vi "CANOpen_Get Section References by GUID for NMT.vi"(7 "Nodes":T2[](array[typedef]) {"NMT"."Node init static SDO state" items=["start remote node"=1, "enter pre-operational"=128]; "NMT"."Node run state" items=["start remote node"=1, "stop remote node"=2, "enter pre-operational"=128, "reset node"=129, "reset communication"=130]; "Dynamic SDOs"."Block Data" format="%.0x"; "RPDOs"."PDO Channel" items=["PDO 1", "PDO 2", "PDO 3", "PDO 4"]; "RPDOs"."Parameters"."Bit Offset" max=8 step=1; "RPDOs"."Parameters"."Byte Offset" max=8 step=1; "TPDOs"."PDO Channel" items=["PDO 1", "PDO 2", "PDO 3", "PDO 4"]; "TPDOs"."Parameters"."Bit Offset" max=8 step=1; "TPDOs"."Parameters"."Byte Offset" max=8 step=1; "SDOs"."Block Data" format="%.0x"}, 8 "error in (no error)":errorcluster, 10 "Node Refs":T1[](array[typedef]) format="%.0x", 11 "Device Ref":T1 format="%.0x") -> (0 "error out":errorcluster, 2 "Data References":T11 {"Hardware Output"."Channel Pairs"."Chan Refs"."Data Reference" format="%.0x"; "Hardware Input"."Channel Pairs"."Chan Refs" format="%.0x"}, 3 "Device Ref out":T1=18446744073709551615 format="%.0x")   [LabVIEW 2013, in "CANOpen Addon Custom Device.lvlib"]
uses:
  CANOpen Addon Custom Device.lvlib
  <vilib>/NI Veristand/Custom Device API/Custom Device Item Ref.ctl
  CANOpen_VS Status Management Data Refs.ctl
  Async VIs/CANOpen_Main/SubVIs/CanOpen_NMT_HWOut_ChannelPairs.ctl
  <vilib>/NI Veristand/Custom Device API/Block Data Reference.ctl
  <vilib>/NI Veristand/Custom Device API/Data Reference.ctl
  Async VIs/CANOpen_Main/SubVIs/CanOpen_NMT_HWIn_ChannelPairs.ctl
  CANOpen_Node Message Settings.ctl
  Shared Code/CANOpen_PDO Settings.ctl
  Shared Code/CANOpen_PDO Parameter Settings.ctl
  Shared Code/CANOpen_PDO Data Type.ctl
  System Explorer/SubVIs/CANopen Byte Order.ctl
  Shared Code/CANOpen_SDO Settings.ctl
  CANOpen_NMT Settings.ctl
  Async VIs/CANOpen_Main/SubVIs/CanOpen_NMT_Config.ctl
  Async VIs/CANOpen_Main/SubVIs/CanOpen_NMT_Static detect.ctl
  Shared Code/CANOpen Addon GUID Lookup Global.vi
  <vilib>/NI Veristand/Custom Device Tools/Custom Device Utility Library/NI VeriStand - Search for All Items by GUID.vi
  <vilib>/NI Veristand/Custom Device Tools/Custom Device Utility Library/NI VeriStand - Search for Item by GUID.vi
  <vilib>/NI Veristand/Custom Device API/NI VeriStand - Get Channel Data Reference.vi
  <vilib>/NI Veristand/Custom Device API/NI VeriStand - Get Channel Block Data References.vi
  <vilib>/NI Veristand/Custom Device API/Custom Device API.lvlib
  <vilib>/NI Veristand/Custom Device Tools/Custom Device Utility Library/Custom Device Utility Library.lvlib
panel:
  # "LSB"
  # "MSB"
  # "LSB"
  # "MSB"
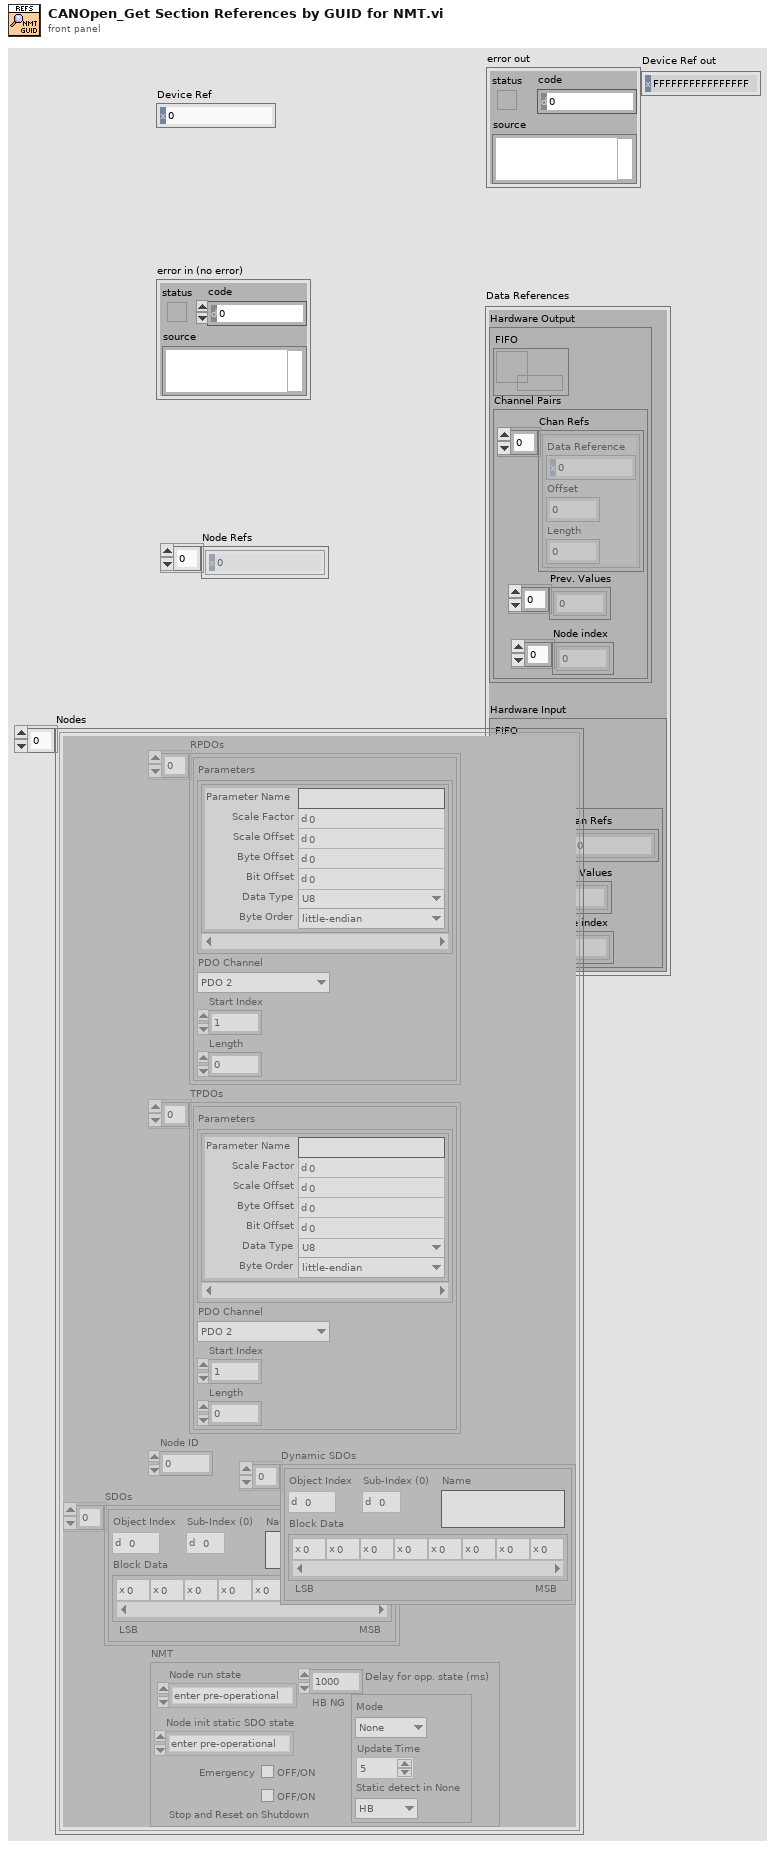
[diagram p1: front panel]
types:
  T1 = typedef "Custom Device API.lvlib/Custom Device Item Ref.ctl" = u64
  T2 = typedef "CANOpen_Node Message Settings.ctl" = cluster{"RPDOs":T3[], "TPDOs":T3[], "Node ID":u8, "SDOs":T7[], "Dynamic SDOs":T7[], "NMT":T8}
  T3 = typedef "CANOpen Addon Custom Device.lvlib/CANOpen_PDO Settings.ctl" = cluster{"Parameters":T4[], "PDO Channel":u8, "Start Index":u32, "Length":u32}
  T4 = typedef "CANOpen Addon Custom Device.lvlib/CANOpen_PDO Parameter Settings.ctl" = cluster{"Parameter Name":string, "Scale Factor":dbl, "Scale Offset":dbl, "Byte Offset":u8, "Bit Offset":u8, "Data Type":T5, "Byte Order":T6}
  T5 = typedef "CANOpen Addon Custom Device.lvlib/CANOpen_PDO Data Type.ctl" = enum16{"U8", "U16", "U32", "I8", "I16", "I32", "Single", "Double", "Boolean"}
  T6 = typedef "CANOpen Addon Custom Device.lvlib/CANopen Byte Order.ctl" = enum16{"big-endian network order", "little-endian"}
  T7 = typedef "CANOpen Addon Custom Device.lvlib/CANOpen_SDO Settings.ctl" = cluster{"Object Index":u16, "Sub-Index (0)":u8, "Block Data":u8[], "Name":string}
  T8 = typedef "CANOpen Addon Custom Device.lvlib/CANOpen_NMT Settings.ctl" = cluster{"Node run state":u16, "Emergency":bool, "HB NG":T9, "Delay for opp. state (ms)":dbl, "Node init static SDO state":u16, "Stop and Reset on Shutdown":bool}
  T9 = typedef "CANOpen Addon Custom Device.lvlib/CanOpen_NMT_Config.ctl" = cluster{"Mode":T10, "Update Time":u16, "Static detect in None":T10}
  T10 = typedef "CANOpen Addon Custom Device.lvlib/CanOpen_NMT_Static detect.ctl" = enum16{"None", "HB", "NG"}
  T11 = typedef "CANOpen Addon Custom Device.lvlib/CANOpen_VS Status Management Data Refs.ctl" = cluster{"Hardware Output":cluster{"FIFO":refnum<k33>, "Channel Pairs":T12}, "Hardware Input":cluster{"FIFO":refnum<k33>, "Channel Pairs":T15}}
  T12 = typedef "CANOpen Addon Custom Device.lvlib/CanOpen_NMT_HWOut_ChannelPairs.ctl" = cluster{"Chan Refs":T13[], "Prev. Values":dbl[], "Node index":dbl[]}
  T13 = typedef "Custom Device API.lvlib/Block Data Reference.ctl" = cluster{"Data Reference":T14, "Offset":i32, "Length":i32}
  T14 = typedef "Custom Device API.lvlib/Data Reference.ctl" = i32
  T15 = typedef "CANOpen Addon Custom Device.lvlib/CanOpen_NMT_HWIn_ChannelPairs.ctl" = cluster{"Chan Refs":T14[], "Prev. Values":dbl[], "Node index":dbl[]}
  T16 = typedef "Custom Device API.lvlib/Custom Device Item Info.ctl" = cluster{"Name":string, "Is Channel":bool, "GUID":string, "Is Waveform":bool}
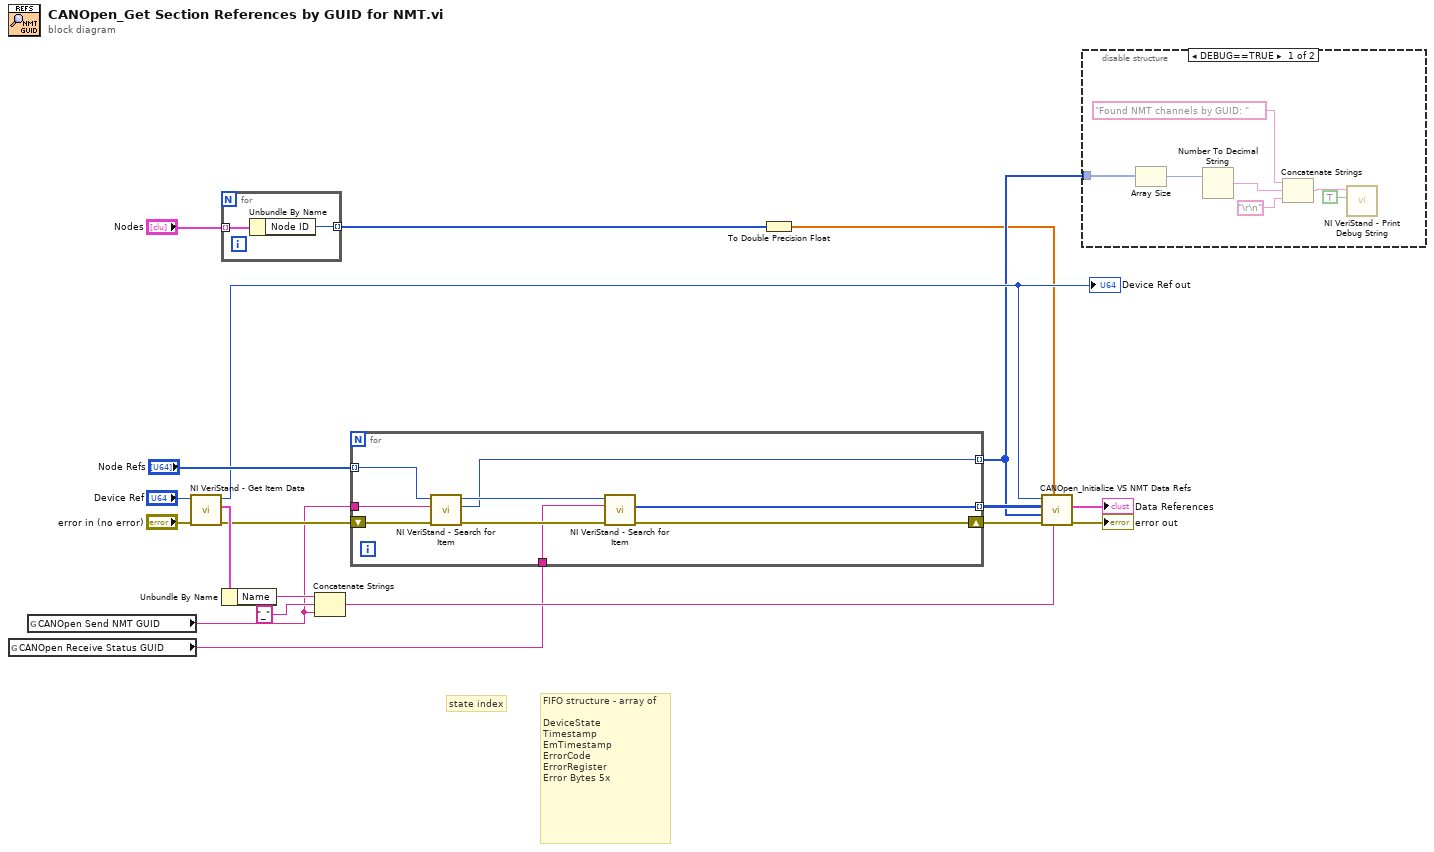
[diagram p0: block diagram]
diagram:
  # "state index"
  # "FIFO structure - array of\n\nDeviceState\nTimestamp\nEmTimestamp\nErrorCode\nErrorRegister\nError Bytes 5x"
  n1 = global read "CANOpen Addon GUID Lookup Global.vi" "CANOpen Receive Status GUID"() -> (w7:string)
  n2 = global read "CANOpen Addon GUID Lookup Global.vi" "CANOpen Send NMT GUID"() -> (w10:string)
  n3 = call <vilib>:"NI VeriStand - Get Item Data.vi"("error in (no error)"="error in (no error)", "Item Ref in"="Device Ref") -> ("error out"=w12:errorcluster, "Item Info"=w19:T16, "Item Ref out"=w6:T1)  [unwired: 6 in, 1 out]
  "Device Ref out" <- w6
  n4 = for {
    tunnel: "Nodes" -> [w21] mode=indexing
    tunnel: [w20] -> w2 mode=indexing
    n5 = Unbundle By Name(w21) -> ("Node ID"=w20:u8)
  }
  n6 = Unbundle By Name(w19) -> ("Name"=w16:string)
  n7 = Concatenate Strings(w16, "_" ("string"), w10) -> (w9:string)
  n8 = for {
    tunnel: w10 -> [w30]
    shift-right: [w24] -> w11
    shift-left: w12 -> [w26]
    tunnel: "Node Refs" -> [w25] mode=indexing
    tunnel: [w23] -> w4 mode=indexing
    tunnel: w7 -> [w27]
    tunnel: [w22] -> w5 mode=indexing
    n9 = call-poly <vilib>:"NI VeriStand - Search for Item.vi"("error in"=w26, "Item GUID"=w30, "Section Ref in"=w25) -> ("error out"=w28:errorcluster, "Item Ref"=w23:T1, "Section Ref out"=w29:T1)  [unwired: 5 in, 1 out]
    n10 = call-poly <vilib>:"NI VeriStand - Search for Item.vi"("error in"=w28, "Item GUID"=w27, "Section Ref in"=w29) -> ("error out"=w24:errorcluster, "Item Refs"=w22:T1[])  [unwired: 5 in, 2 out]
  }
  n11 = To Double Precision Float(number=w2) -> (double precision float=w1:dbl[])
  n12 = call "CANOpen_Initialize VS NMT Data Refs.vi"("Name"=w9, "Node indexes"=w1, "error in (no error)"=w11, "Hardware Output Refs"=w4, "Hardware Input Refs"=w5, "Device Ref"=w6) -> ("error out"=→"error out":errorcluster, "Data References"=→"Data References":T11)  [unwired: 4 in]
  n13 = disable-structure shown="DEBUG==TRUE" {
    disable-tunnel: w4 -> [w35 _]
    frame condition #0 {
      n14 = Array Size(array=w35) -> (size(s)=w34:i32)
      n15 = Number To Decimal String(number=w34) -> (decimal integer string=w33:string)  [unwired: 1 in]
      n16 = Concatenate Strings("Found NMT channels by GUID: " ("string"), w33, "\r\n") -> (w37:string)
      n17 = call <vilib>:"NI VeriStand - Print Debug String.vi"("Add to log file? (T)"=TRUE, "Message"=w37) -> ()  [unwired: 9 in, 1 out]
    }
    frame condition #1 (active) {
    }
  }
